vi "get selected list item.vi"(8 "error in (no error)":errorcluster, 11 "ListBox in":refnum<vi>) -> (0 "error out":errorcluster, 2 "valid selection?":bool, 3 "element name":string)   [LabVIEW 2014, in "Shared Memory editor node.lvclass"]
uses:
  Shared Memory editor node.lvclass
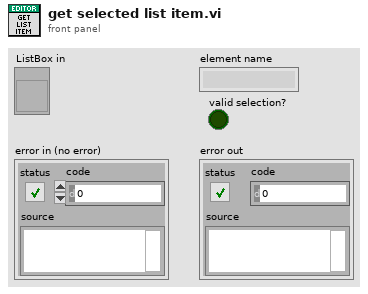
[diagram p1: front panel]
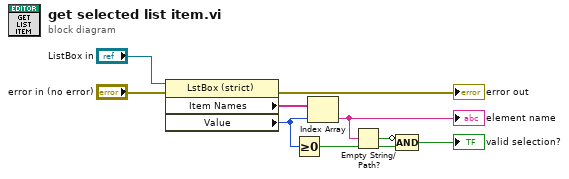
[diagram p0: block diagram]
diagram:
  n1 = property class="LstBox (strict)"(reference="ListBox in", error in="error in (no error)") -> (error out=→"error out":errorcluster, "Item Names"=w2:string[], "Value"=w3:i32)  [unwired: 1 out]
  n2 = Greater Or Equal To 0?(x=w3) -> (x >= 0?=w4:bool)
  n3 = Index Array(array=w2, index=w3) -> (element=w5:string)
  "element name" <- w5
  n4 = Empty String/Path?(string/path=w5) -> (empty?=w6:bool)
  n5 = Compound Arithmetic op=AND(invert w6, w4) -> (→"valid selection?":bool)
